vi "Example Configuration.vi"() -> ()   [LabVIEW 2010]
uses:
  C:/tf/play/labview/Tinkerforge.dll
  Tinkerforge.dll
panel:
  in  "stop":bool
  in  "uid":string="63oL6P"
  in  "port":i32=4223
  in  "host":string="localhost"
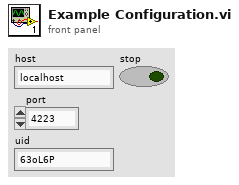
[diagram p1: front panel]
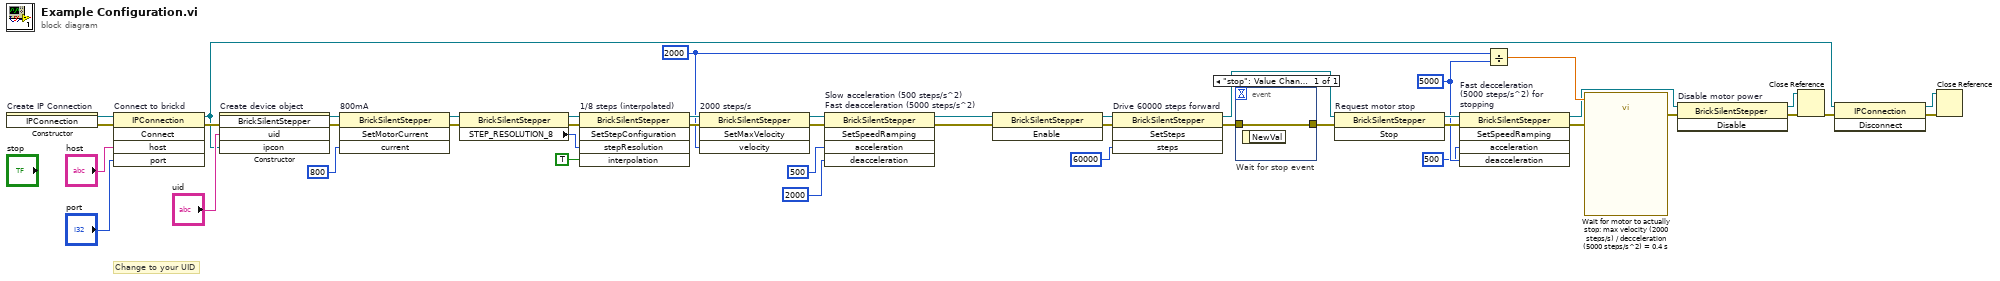
[diagram p0: block diagram]
diagram:
  w9 = 5000 ("deacceleration")
  w1 = 2000 ("velocity")
  # "Change to your UID"
  n1 = constructor on="Create IP Connection" class="IPConnection"() -> (reference out=w44:refnum<k24>, error out=w22:errorcluster)  [unwired: 3 in, 1 out]
  n2 = invoke on="Connect to brickd" class="IPConnection" method="Connect"(reference=w44, error in=w22, "host"="host", "port"="port") -> (reference out=w35:refnum<k24>, error out=w40:errorcluster)  [unwired: 1 in, 3 out]
  n3 = constructor on="Create device object" class="BrickSilentStepper"(error in=w40, "uid"="uid", "ipcon"=w35) -> (reference out=w38:refnum<k24>, error out=w39:errorcluster)  [unwired: 2 in, 3 out]
  n4 = invoke on="800mA" class="BrickSilentStepper" method="SetMotorCurrent"(reference=w38, error in=w39, "current"=800) -> (reference out=w20:refnum<k24>, error out=w19:errorcluster)  [unwired: 1 in, 2 out]
  n5 = property class="BrickSilentStepper"(reference=w20, error in=w19) -> (reference out=w21:refnum<k24>, error out=w18:errorcluster, "STEP_RESOLUTION_8"=w17:u8)
  n6 = invoke on="1/8 steps (interpolated)" class="BrickSilentStepper" method="SetStepConfiguration"(reference=w21, error in=w18, "stepResolution"=w17, "interpolation"=TRUE) -> (reference out=w31:refnum<k24>, error out=w32:errorcluster)  [unwired: 1 in, 3 out]
  n7 = invoke on="2000 steps/s" class="BrickSilentStepper" method="SetMaxVelocity"(reference=w31, error in=w32, "velocity"=w1) -> (reference out=w29:refnum<k24>, error out=w30:errorcluster)  [unwired: 1 in, 2 out]
  n8 = invoke on="Slow acceleration (500 steps/s^2)\nFast deacceleration (5000 steps/s^2)" class="BrickSilentStepper" method="SetSpeedRamping"(reference=w29, error in=w30, "acceleration"=500, "deacceleration"=2000) -> (reference out=w26:refnum<k24>, error out=w27:errorcluster)  [unwired: 1 in, 3 out]
  n9 = invoke class="BrickSilentStepper" method="Enable"(reference=w26, error in=w27) -> (reference out=w24:refnum<k24>, error out=w25:errorcluster)  [unwired: 1 in, 1 out]
  n10 = invoke on="Drive 60000 steps forward" class="BrickSilentStepper" method="SetSteps"(reference=w24, error in=w25, "steps"=60000) -> (reference out=w5:refnum<k24>, error out=w6:errorcluster)  [unwired: 1 in, 2 out]
  n11 = event "Wait for stop event" shown="[0] \"stop\": Value Change" {
    selector: _ -> [_]
    dyn-events: _ -> [_]
    timeout: _ -> [_]
    tunnel: [w45] -> w7
    tunnel: w6 -> [w45]
    event "stop": Value Change {
      n12 = event-data() -> ()  [unwired: 1 in, 1 out]
    }
  }
  n13 = invoke on="Request motor stop" class="BrickSilentStepper" method="Stop"(reference=w5, error in=w7) -> (reference out=w13:refnum<k24>, error out=w11:errorcluster)  [unwired: 1 in, 1 out]
  n14 = invoke on="Fast decceleration\n(5000 steps/s^2) for\nstopping" class="BrickSilentStepper" method="SetSpeedRamping"(reference=w13, error in=w11, "acceleration"=500, "deacceleration"=w9) -> (reference out=w12:refnum<k24>, error out=w10:errorcluster)  [unwired: 1 in, 3 out]
  n15 = Divide(x=w1, y=w9) -> (x/y=w14:dbl)
  n16 = call "Wait for motor to actually stop: max velocity (2000 steps/s) / decceleration (5000 steps/s^2) = 0.4 s"("error in (no error)"=w10, "Delay Time (s)"=w14) -> ("error out"=w15:errorcluster)  [unwired: 9 in]
  n17 = invoke on="Disable motor power" class="BrickSilentStepper" method="Disable"(reference=w12, error in=w15) -> (reference out=w3:refnum<k24>, error out=w4:errorcluster)  [unwired: 1 in, 1 out]
  n18 = Close Reference(reference=w3, error in (no error)=w4) -> (error out=w37:errorcluster)
  n19 = invoke class="IPConnection" method="Disconnect"(reference=w35, error in=w37) -> (reference out=w34:refnum<k24>, error out=w36:errorcluster)  [unwired: 1 in, 1 out]
  n20 = Close Reference(reference=w34, error in (no error)=w36) -> ()  [unwired: 1 out]
